vi "create scan vectr2.vi"(3 "Table Control":string[][](table)) -> (0 "parameters":dbl[](array[numeric]), 2 "positions":dbl[](array[numeric]))   [LabVIEW 2019]
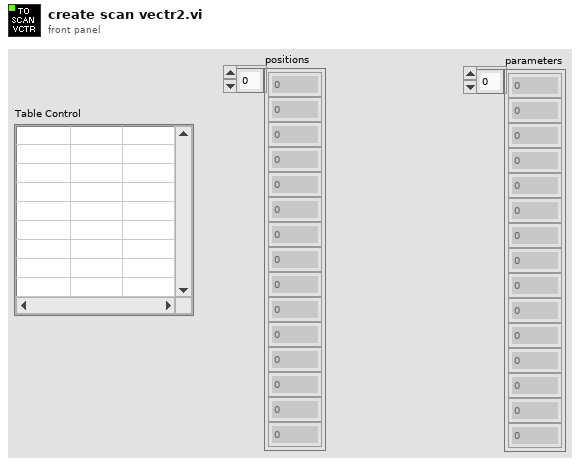
[diagram p1: front panel]
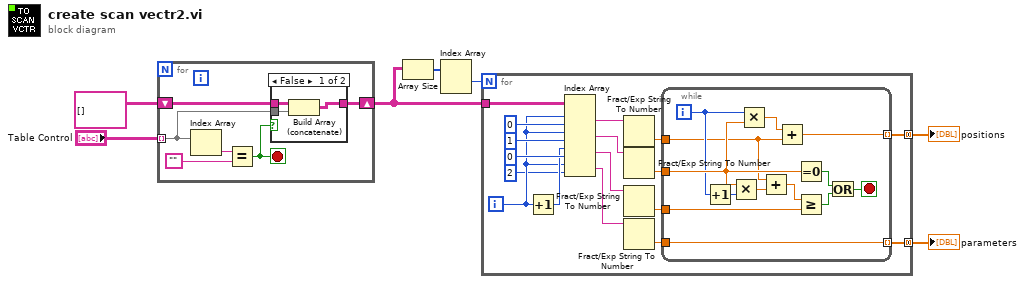
[diagram p0: block diagram]
diagram:
  n1 = for {
    tunnel: "Table Control" -> [w9] mode=indexing
    shift-right: [w8] -> w4
    shift-left: string[][] [] ("t") -> [w11]
    stop <- w10 stop-if-true
    n2 = Index Array(array=w9) -> (element=w12:string)  [unwired: 1 in]
    n3 = Equal?(x=w12, y="") -> (x = y?=w10:bool)
    n4 = case shown="False" w10 {
      tunnel: w11 -> [w16 w17]
      tunnel: w9 -> [w15 _]
      tunnel: [w14 w17] -> w8
      frame False {
        n5 = Build Array (concatenate)(w16, w15) -> (w14:string[][])
      }
      frame True {
      }
    }
  }
  n6 = Array Size(array=w4) -> (size(s)=w3:i32[])
  n7 = Index Array(array=w3) -> (element #1=w2:i32)  [unwired: 2 in, 1 out]
  n8 = for {
    N: w2 -> [_]
    tunnel: w4 -> [w30]
    tunnel: [w23] -> w5 mode=concatenating
    tunnel: [w18] -> w1 mode=concatenating
    i -> [w22]
    n9 = Increment(x=w22) -> (x+1=w32:i32)
    n10 = Index Array(array=w30, index (row) #1=w22, index (col) #1=0 ("disabled index (col)"), index (row) #2=w22, index (col) #2=1 ("disabled index (col)"), index (row) #3=w32, index (col) #3=0 ("disabled index (col)"), index (row) #4=w22, index (col) #4=2 ("disabled index (col)")) -> (element #1=w29:string, element #2=w28:string, element #3=w27:string, element #4=w20:string)
    n11 = Fract/Exp String To Number(string=w29) -> (number=w26:dbl)  [unwired: 3 in, 1 out]
    n12 = Fract/Exp String To Number(string=w28) -> (number=w25:dbl)  [unwired: 3 in, 1 out]
    n13 = Fract/Exp String To Number(string=w27) -> (number=w24:dbl)  [unwired: 3 in, 1 out]
    n14 = Fract/Exp String To Number(string=w20) -> (number=w19:dbl)  [unwired: 3 in, 1 out]
    n15 = while {
      tunnel: w26 -> [w37]
      tunnel: w25 -> [w39]
      tunnel: w24 -> [w43]
      tunnel: [w47] -> w23 mode=indexing
      tunnel: w19 -> [w35]
      tunnel: [w35] -> w18 mode=indexing
      i -> [w38]
      stop <- w40 stop-if-true
      n16 = Increment(x=w38) -> (x+1=w45:i32)
      n17 = Multiply(x=w39, y=w45) -> (x*y=w46:dbl)
      n18 = Multiply(x=w38, y=w39) -> (x*y=w36:dbl)
      n19 = Add(x=w37, y=w46) -> (x+y=w44:dbl)
      n20 = Add(x=w36, y=w37) -> (x+y=w47:dbl)
      n21 = Equal To 0?(x=w39) -> (x = 0?=w42:bool)
      n22 = Greater Or Equal?(x=w44, y=w43) -> (x >= y?=w41:bool)
      n23 = Or(x=w42, y=w41) -> (x .or. y?=w40:bool)
    }
  }
  "positions" <- w5
  "parameters" <- w1
